vi "main.vi"() -> ()   [LabVIEW 2016]
uses:
  controls/Level2.ctl
panel:
  in  "StringArray":string[](array[string])
  in  "BooleanArray":bool[](array[boolean])
  in  "NumericArray":dbl[](array[numeric])
  in  "BigCluster":T2
  in  "Cluster":T3
  in  "String":string
  in  "Boolean":bool
  in  "Numeric":dbl
  in  "Tab Control":T4(tab)
  in  "BigCluster":T2
  in  "Cluster":T3
  in  "String":string
  in  "Boolean":bool
  in  "Numeric":dbl
  in  "Time lapse(sec)":u32
  in  "Panel Name":string
  in  "Refresh":bool
  in  "Listbox":i32(listbox)
  in  "Panel Name 2":string
  in  "Listbox 2":i32(listbox)
  in  "Run":bool
  in  "DisableListbox":i32(listbox)
  in  "MultiselectListbox":i32[](listbox)
  in  "Single Listbox":i32(listbox)
  out "Listbox Value":i32
  out "Selected Value":i32[](array[numeric])
  in  "Disabled MC Listbox":i32(listbox)
  in  "Multiselect MC Listbox":i32[](listbox)
  in  "MC Listbox":i32(listbox)
  out "MCListbox Value":i32
  out "MCL Selected Value":i32[](array[numeric])
  in  "OK":bool
  in  "Stop":bool
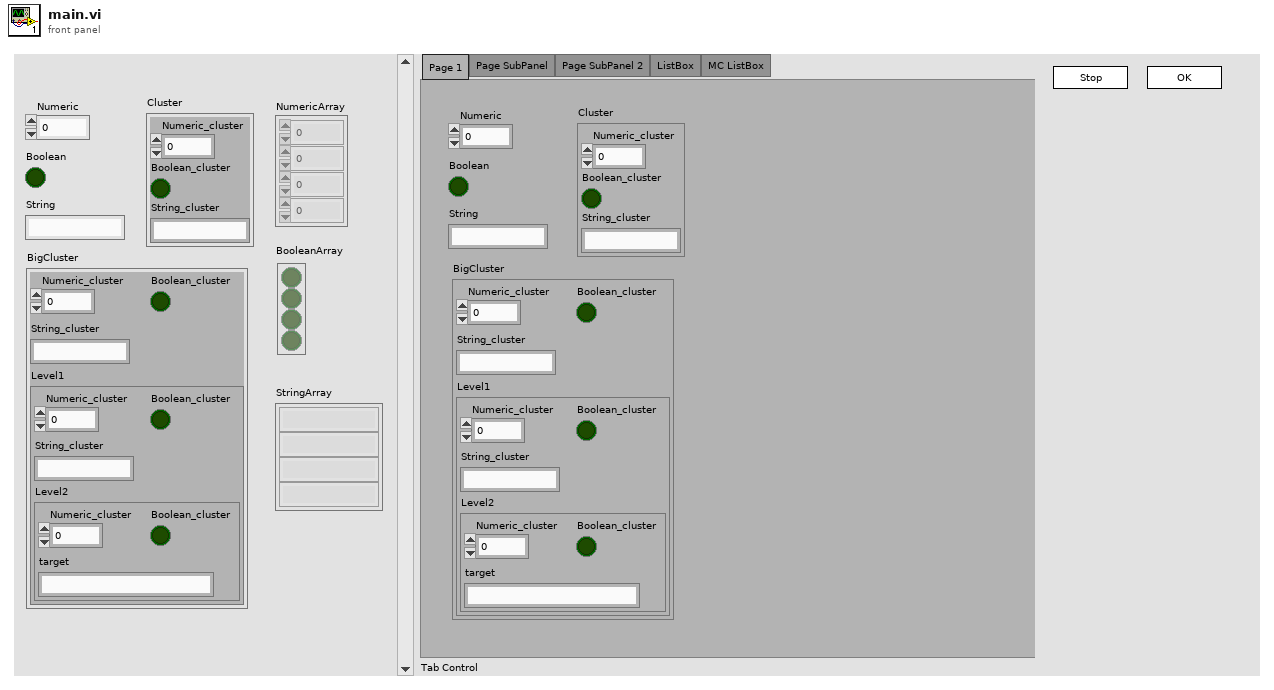
[diagram p1: front panel]
types:
  T1 = typedef "Level2.ctl" = cluster{"Numeric_cluster":dbl, "Boolean_cluster":bool, "target":string}
  T2 = cluster{"Numeric_cluster":dbl, "Boolean_cluster":bool, "String_cluster":string, "Level1":cluster{"Numeric_cluster":dbl, "Boolean_cluster":bool, "String_cluster":string, "Level2":T1}}
  T3 = cluster{"Numeric_cluster":dbl, "Boolean_cluster":bool, "String_cluster":string}
  T4 = enum32{"Page 1", "Page SubPanel", "Page SubPanel 2", "ListBox", "MC ListBox"}
  T5 = enum32{"Invalid", "Standard", "Closed", "Hidden", "Minimized", "Maximized"}
  T6 = enum32{"invalid app kind", "Development System", "Run Time System", "Student Edition", "Embedded LabVIEW", "Evaluation", "Custom"}
  T7 = enum8{"Enabled", "Disabled", "Disabled and Grayed Out"}
  T8 = cluster{"Core":cluster{"Current VI Reference":refnum<vi>, "Close Panel on Exit?":bool}, "VI Name":string, "VI Ref":refnum<vi>, "Panel Folder Path":path, "Time lapse(sec)":u32, "Panel 2 Folder Path":path, "Panel 2 VI ref":refnum<vi>, "VI Running?":bool}
  T9 = cluster{"Current VI Reference":refnum<vi>, "Close Panel on Exit?":bool}
  T10 = enum32{"Bad", "Idle", "Run top level", "Running"}[]
  T11 = enum32{"Bad", "Idle", "Run top level", "Running"}
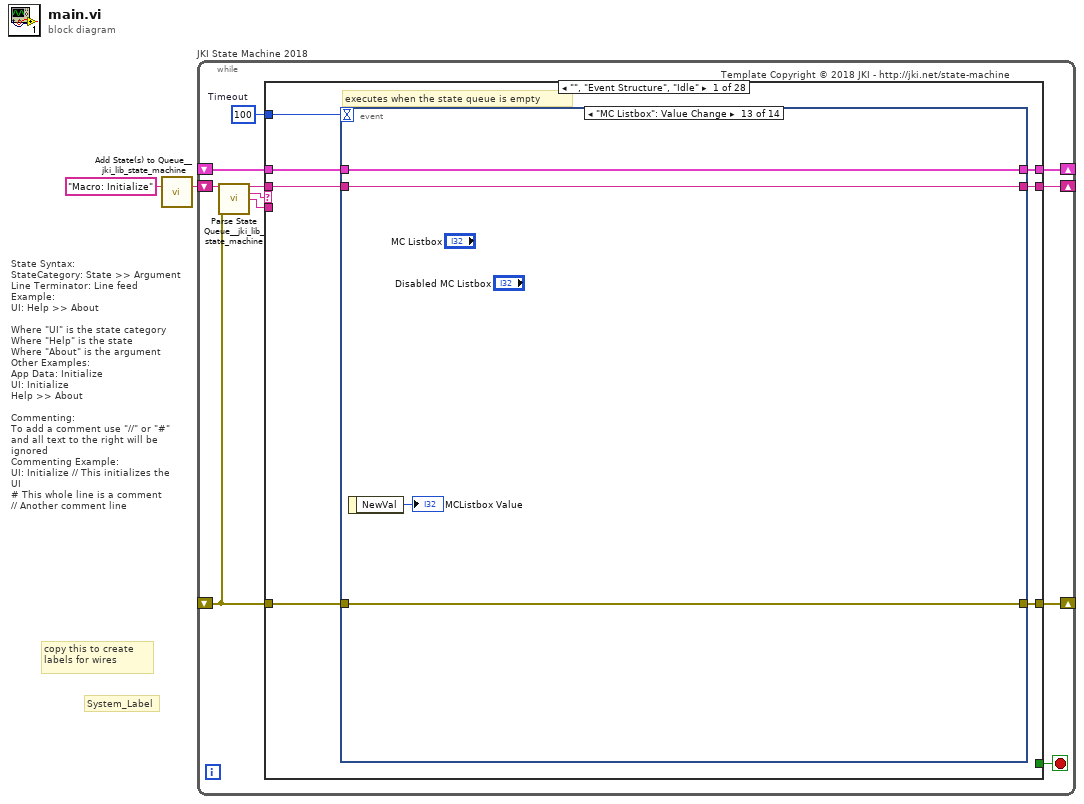
[diagram p0: block diagram]
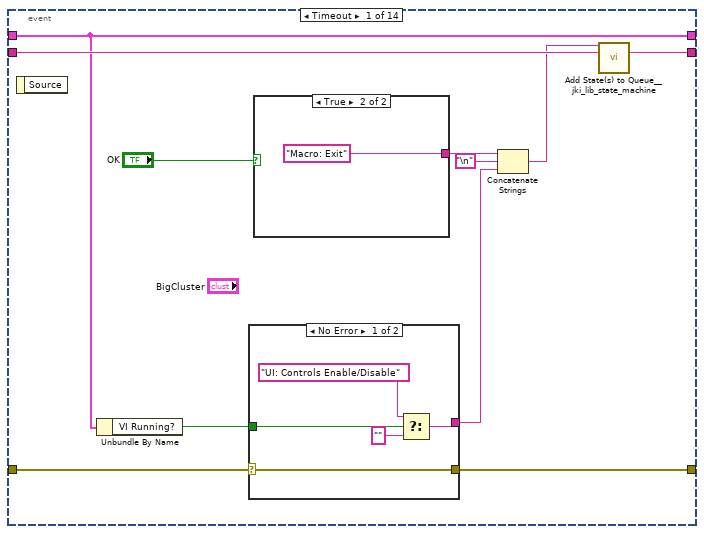
[diagram p2: hidden frame]
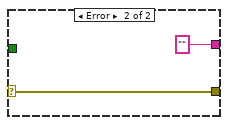
[diagram p3: hidden frame]
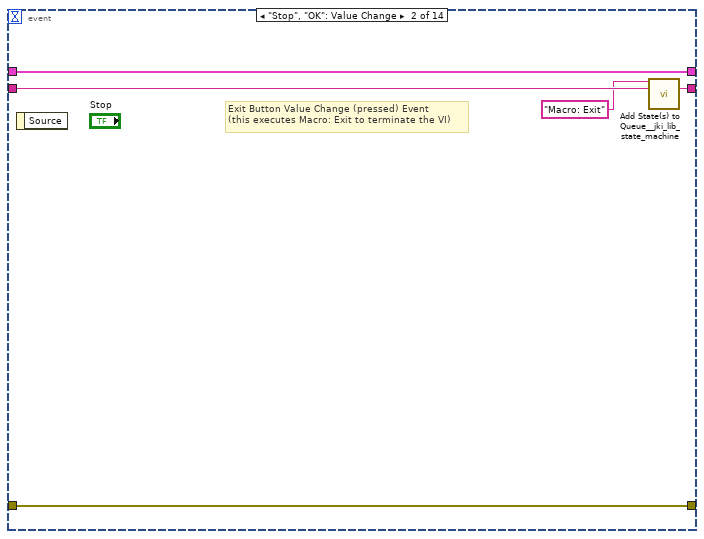
[diagram p5: hidden frame]
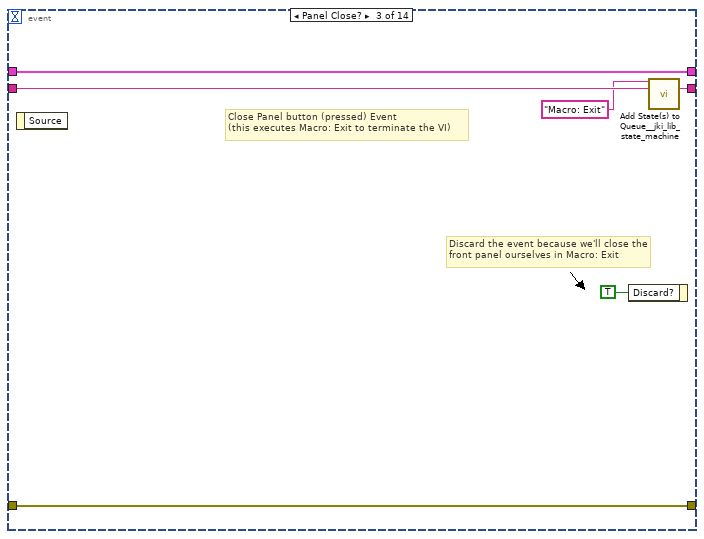
[diagram p6: hidden frame]
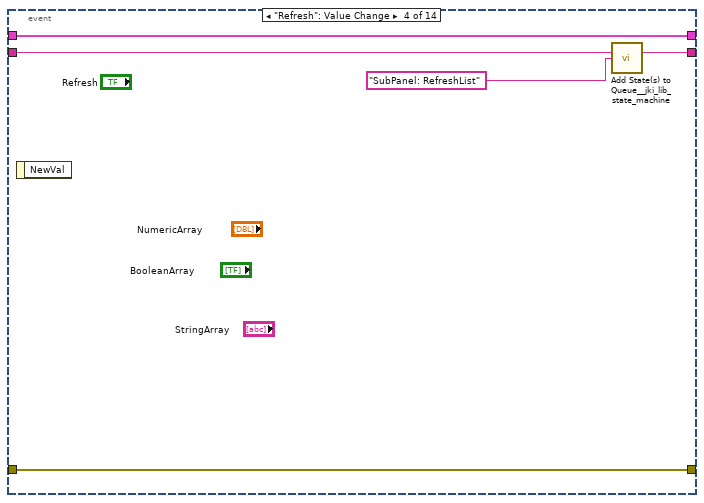
[diagram p7: hidden frame]
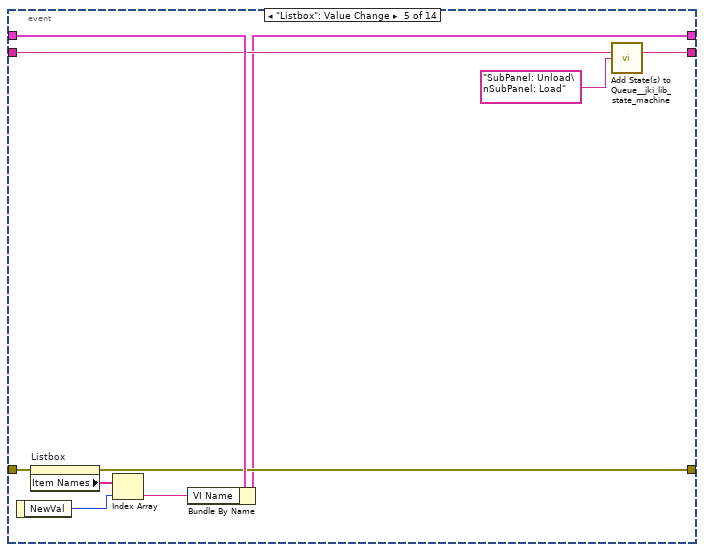
[diagram p8: hidden frame]
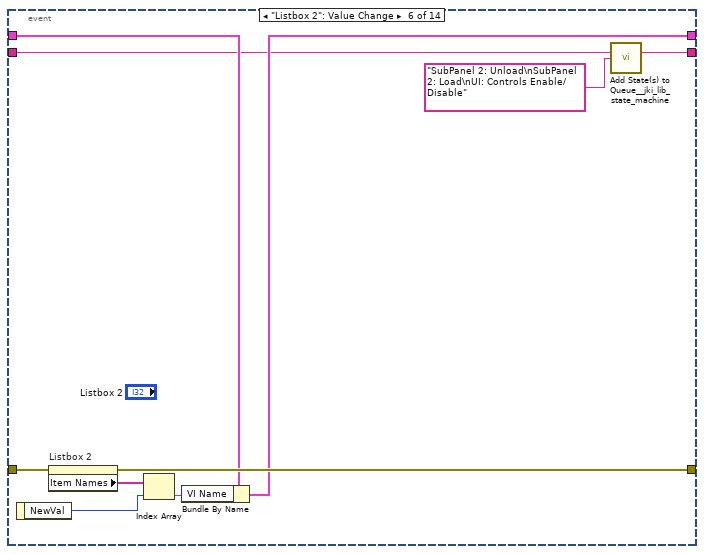
[diagram p9: hidden frame]
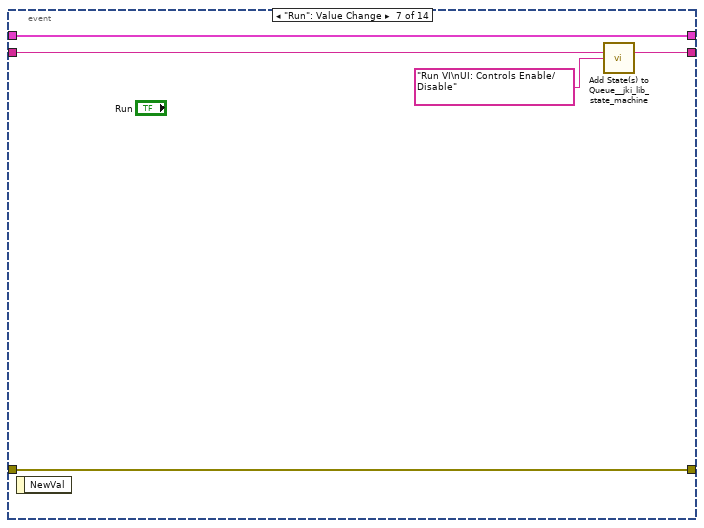
[diagram p10: hidden frame]
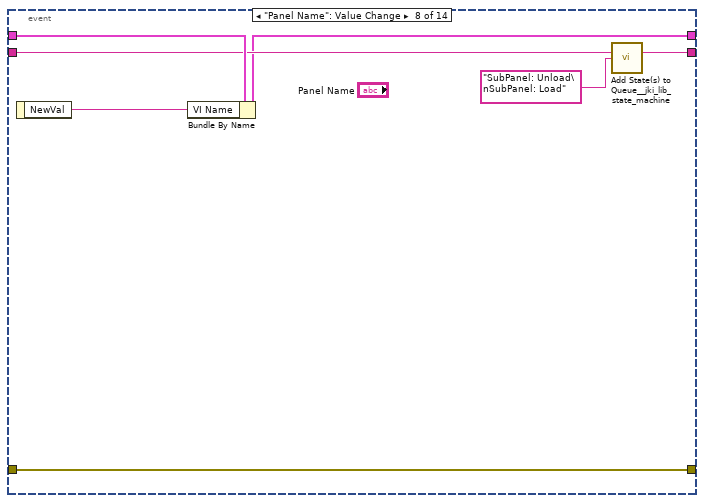
[diagram p11: hidden frame]
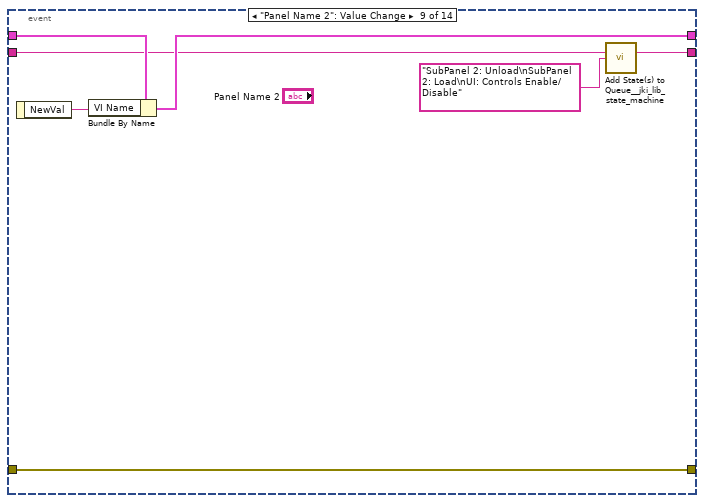
[diagram p12: hidden frame]
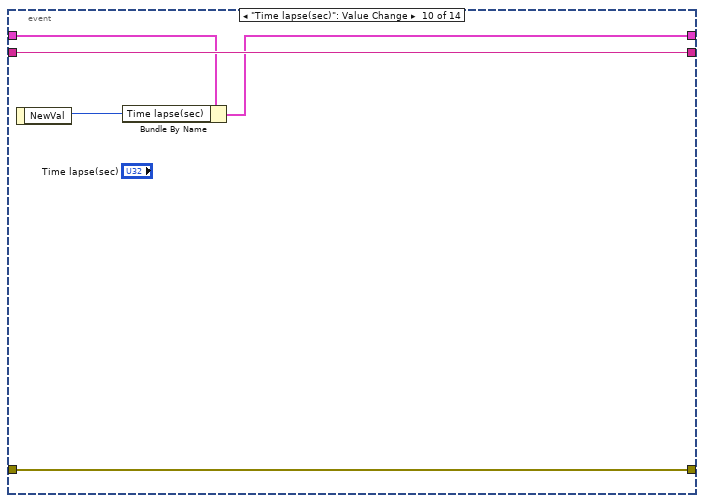
[diagram p13: hidden frame]
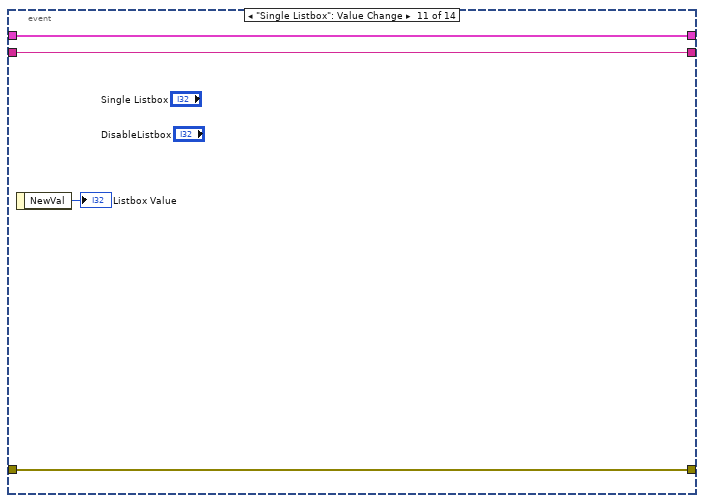
[diagram p14: hidden frame]
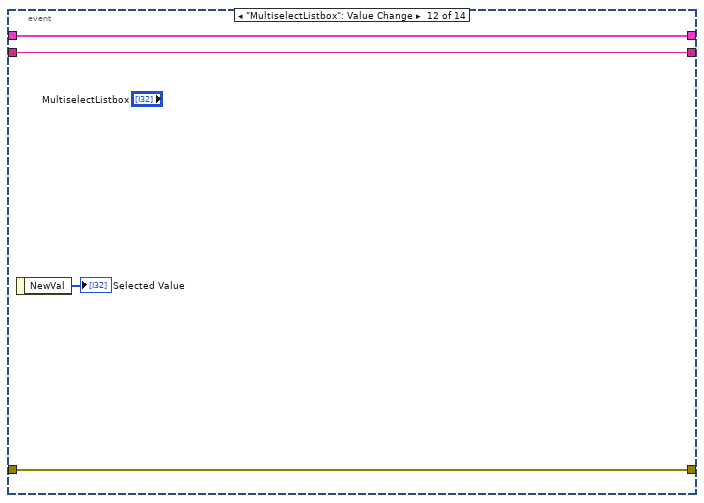
[diagram p15: hidden frame]
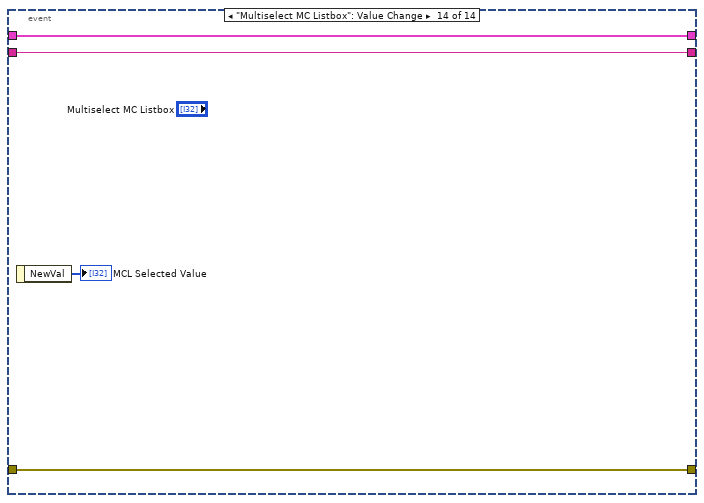
[diagram p16: hidden frame]
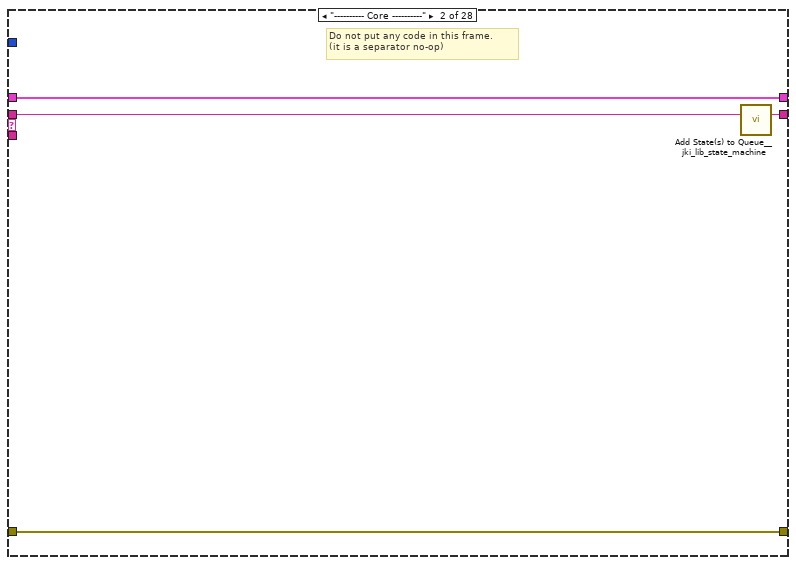
[diagram p17: hidden frame]
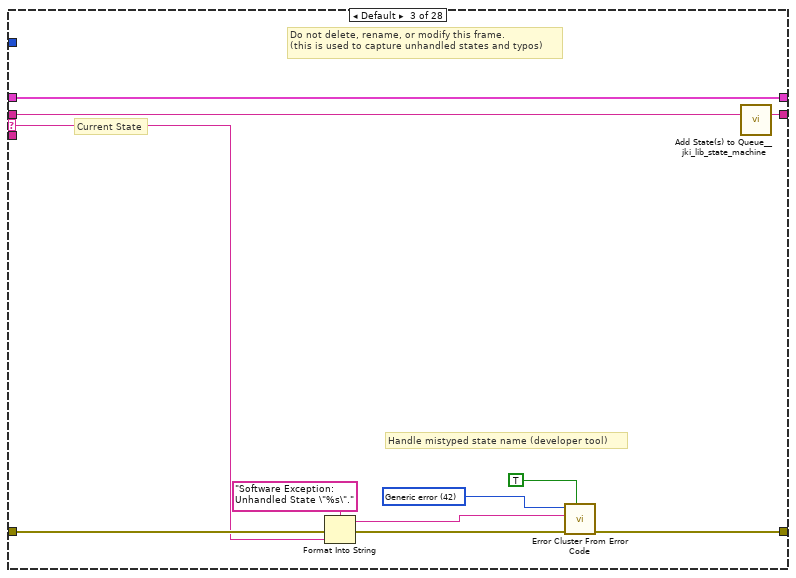
[diagram p18: hidden frame]
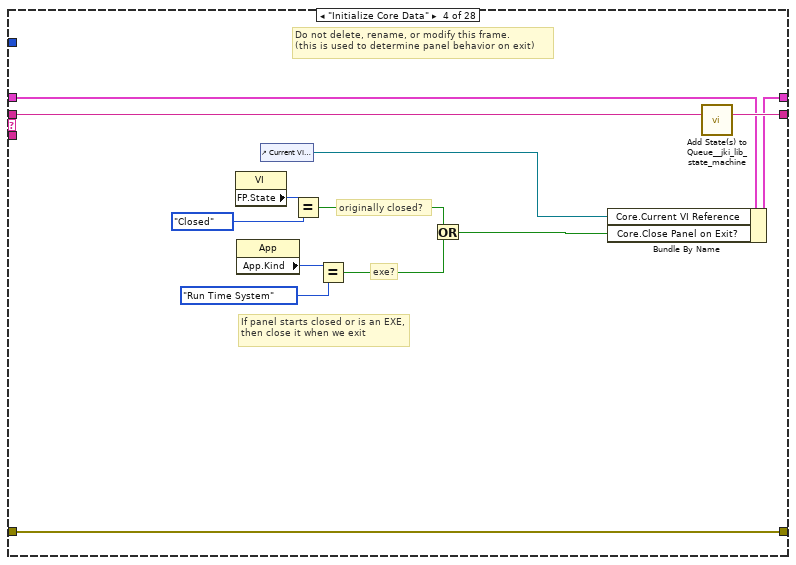
[diagram p19: hidden frame]
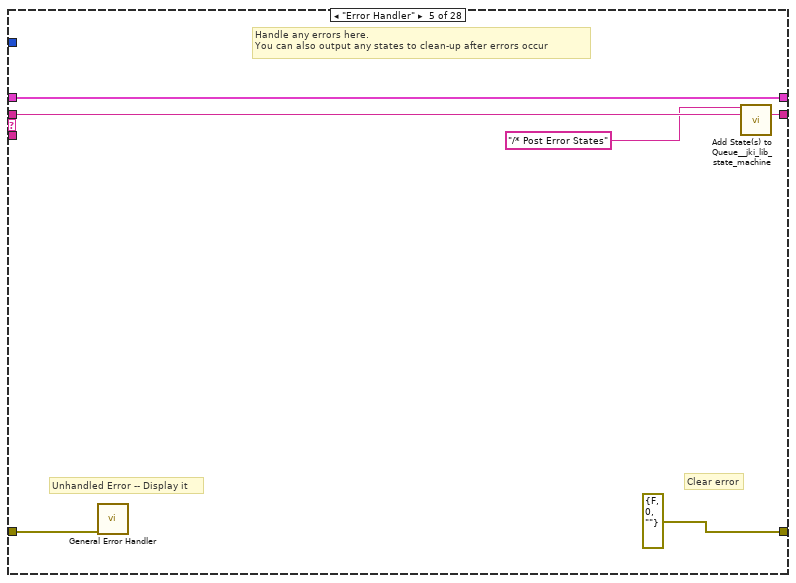
[diagram p20: hidden frame]
diagram:
  # "State Syntax:\nStateCategory: State >> Argument\nLine Terminator: Line feed\nExample:\nUI: Help >> About\n\nWhere \"UI\" is the state category\nWhere \"Help\" is the state\nWhere \"About\" is the argument\nOther Examples:\nApp Data: Initialize\nUI: Initialize\nHelp >> About\n\nCommenting:\nTo add a comment use \"//\" or \"#\" and all text to the right will be ignored\nCommenting Example:\nUI: Initialize // This initializes the UI\n# This whole line is a comment\n// Another comment line"
  # "copy this to create labels for wires"
  # "System_Label"
  n1 = call <vilib>:"Add State(s) to Queue__jki_lib_state_machine.vi"("State(s) in (\"\")"="Macro: Initialize") -> ("States Out"=w2:string)  [unwired: 14 in]
  n2 = while "JKI State Machine 2018" {
    shift-right: [w6] -> _
    shift-left: _ -> [w5]
    shift-right: [w9] -> _
    shift-left: _ -> [w3]
    shift-right: [w8] -> _
    shift-left: w2 -> [w10]
    stop <- w7 stop-if-true
    w4 = 100  # Timeout
    # "Template Copyright © 2018 JKI - http://jki.net/state-machine"
    n3 = call <vilib>:"Parse State Queue__jki_lib_state_machine.vi"("State Queue"=w10, "Error In (no error)"=w3) -> ("Remaining States"=w12:string, "Current State"=w13:string, "Arguments"=w11:string)  [unwired: 11 in]
    n4 = case shown="\"\", \"Event Structure\", \"Idle\"" w13 {
      selector: w13 -> [_ _ w120 _ _ _ _ _ _ _ _ _ _ _ _ _ _ _ _ _ _ _ _ _ _ _ _ _]
      tunnel: w12 -> [w20 w119 w124 w143 w149 w154 w158 w178 w184 w188 w195 w201 w212 w281 w293 w305 w310 w320 w324 w338 w348 w371 w404 w418 w420 w431 w435 w439]
      tunnel: w11 -> [_ _ _ _ _ _ _ _ _ _ _ w196 w206 _ _ _ _ _ _ _ _ _ _ _ _ _ _ _]
      tunnel: w5 -> [w18 w116 w122 w136 w146 w152 w155 _ w179 w185 w193 w199 w208 w279 w283 w302 w307 w317 w321 w333 w345 w366 w402 w410 w419 w424 w432 w436]
      tunnel: [w17 w117 w126 w140 errorcluster {"status"=FALSE, "code"=0, "source"=""} ("error out") w151 w156 w159 w180 w186 w190 w197 w209 w278 w284 w303 w308 w318 w322 w326 w339 w369 w400 w412 w421 w426 w433 w437] -> w9
      tunnel: w3 -> [w16 w117 w125 w140 w145 w151 w156 w160 w181 w186 w192 w198 w210 w278 w285 w303 w308 w318 w322 w336 w341 w363 w403 w413 w421 w429 w433 w437]
      tunnel: [w19 w118 w123 w142 w148 w153 w157 w177 w183 w187 w194 w200 w211 w280 w293 w304 w309 w319 w323 w337 w347 w370 w404 w418 w420 w431 w434 w438] -> w8
      tunnel: [_ _ _ _ _ TRUE _ _ _ _ _ _ _ _ _ _ _ _ _ _ _ _ _ _ _ _ _ _] -> w7
      tunnel: [w15 w116 w122 w141 w146 w152 w155 w172 w179 w185 w193 w199 w208 w279 w283 w302 w307 w317 w321 w333 w345 w365 w402 w409 w419 w423 w432 w436] -> w6
      tunnel: w4 -> [w14 _ _ _ _ _ _ _ _ _ _ _ _ _ _ _ _ _ _ _ _ _ _ _ _ _ _ _]
      frame "", "Event Structure", "Idle" {
        # "executes when the state queue is empty"
        n5 = event shown="[12] \"MC Listbox\": Value Change" {
          selector: _ -> [_ _ _ _ _ _ _ _ _ _ _ _ _ _]
          dyn-events: _ -> [_ _ _ _ _ _ _ _ _ _ _ _ _ _]
          timeout: w14 -> [_ _ _ _ _ _ _ _ _ _ _ _ _ _]
          tunnel: w20 -> [w31 w44 w50 w53 w64 w67 w78 w86 w89 w99 w103 w107 w111 w115]
          tunnel: [w30 w43 w49 w52 w63 w66 w77 w85 w88 w99 w103 w107 w111 w115] -> w19
          tunnel: w18 -> [w28 w41 w47 w54 w65 w70 w79 w87 w92 w96 w101 w105 w109 w113]
          tunnel: [w21 w42 w48 w55 w60 w73 w80 w83 w94 w98 w102 w106 w110 w114] -> w17
          tunnel: w16 -> [w22 w42 w48 w55 w61 w74 w80 w83 w94 w98 w102 w106 w110 w114]
          tunnel: [w28 w41 w47 w54 w57 w69 w79 w81 w91 w95 w101 w105 w109 w113] -> w15
          event Timeout {
            n6 = event-data() -> ()  [unwired: 1 in, 1 out]
            n7 = Unbundle By Name(w28) -> ("VI Running?"=w27:bool)
            n8 = case shown="No Error" w22 {
              selector: w22 -> [w32 w37]
              tunnel: [w33 ""] -> w26
              tunnel: w27 -> [w36 _]
              tunnel: [w32 w37] -> w21
              frame No Error {
                n9 = Select(t="UI: Controls Enable/Disable", s=w36, f="") -> (s? t:f=w33:string)
              }
              frame Error {
              }
            }
            n10 = case shown="True" "OK" {
              tunnel: [_ "Macro: Exit"] -> w25
              frame False {
              }
              frame True {
              }
            }
            n11 = Concatenate Strings(w25, "\n", w26) -> (w23:string)
            n12 = call <vilib>:"Add State(s) to Queue__jki_lib_state_machine.vi"("State(s) in Front (\"\")"=w23, "State(s) in (\"\")"=w31) -> ("States Out"=w30:string)  [unwired: 13 in]
          }
          event "Stop", "OK": Value Change {
            # "Exit Button Value Change (pressed) Event\n(this executes Macro: Exit to terminate the VI)"
            n13 = event-data() -> ()  [unwired: 1 in, 1 out]
            n14 = call <vilib>:"Add State(s) to Queue__jki_lib_state_machine.vi"("State(s) in Front (\"\")"="Macro: Exit", "State(s) in (\"\")"=w44) -> ("States Out"=w43:string)  [unwired: 13 in]
          }
          event Panel Close? {
            # "Discard the event because we'll close the front panel ourselves in Macro: Exit"
            # "Close Panel button (pressed) Event\n(this executes Macro: Exit to terminate the VI)"
            n15 = event-data() -> ()  [unwired: 1 in, 1 out]
            n16 = event-data("Discard?"=TRUE) -> ()  [unwired: 1 in, 1 out]
            n17 = call <vilib>:"Add State(s) to Queue__jki_lib_state_machine.vi"("State(s) in Front (\"\")"="Macro: Exit", "State(s) in (\"\")"=w50) -> ("States Out"=w49:string)  [unwired: 13 in]
          }
          event "Refresh": Value Change {
            n18 = event-data() -> ()  [unwired: 1 in, 1 out]
            n19 = call <vilib>:"Add State(s) to Queue__jki_lib_state_machine.vi"("State(s) in (\"\")"=w53, "State(s) at Back (\"\")"="SubPanel: RefreshList") -> ("States Out"=w52:string)  [unwired: 13 in]
          }
          event "Listbox": Value Change {
            n20 = event-data() -> ("NewVal"=w58:i32)  [unwired: 1 in]
            n21 = property on="Listbox" class="LstBox (strict)"(error in=w61) -> (error out=w60:errorcluster, "Item Names"=w59:string[])  [unwired: 1 in, 1 out]
            n22 = Index Array(array=w59, index=w58) -> (element=w56:string)
            n23 = Bundle By Name(cluster=w65, "VI Name"=w56) -> (w57:T8)
            n24 = call <vilib>:"Add State(s) to Queue__jki_lib_state_machine.vi"("State(s) in (\"\")"=w64, "State(s) at Back (\"\")"="SubPanel: Unload\nSubPanel: Load") -> ("States Out"=w63:string)  [unwired: 13 in]
          }
          event "Listbox 2": Value Change {
            n25 = event-data() -> ("NewVal"=w72:i32)  [unwired: 1 in]
            n26 = property on="Listbox 2" class="LstBox (strict)"(error in=w74) -> (error out=w73:errorcluster, "Item Names"=w75:string[])  [unwired: 1 in, 1 out]
            n27 = Index Array(array=w75, index=w72) -> (element=w71:string)
            n28 = Bundle By Name(cluster=w70, "VI Name"=w71) -> (w69:T8)
            n29 = call <vilib>:"Add State(s) to Queue__jki_lib_state_machine.vi"("State(s) in (\"\")"=w67, "State(s) at Back (\"\")"="SubPanel 2: Unload\nSubPanel 2: Load\nUI: Controls Enable/Disable") -> ("States Out"=w66:string)  [unwired: 13 in]
          }
          event "Run": Value Change {
            n30 = event-data() -> ()  [unwired: 1 in, 1 out]
            n31 = call <vilib>:"Add State(s) to Queue__jki_lib_state_machine.vi"("State(s) in (\"\")"=w78, "State(s) at Back (\"\")"="Run VI\nUI: Controls Enable/Disable" ("State(s) at Back (\"\")")) -> ("States Out"=w77:string)  [unwired: 13 in]
          }
          event "Panel Name": Value Change {
            n32 = event-data() -> ("NewVal"=w82:string)  [unwired: 1 in]
            n33 = Bundle By Name(cluster=w87, "VI Name"=w82) -> (w81:T8)
            n34 = call <vilib>:"Add State(s) to Queue__jki_lib_state_machine.vi"("State(s) in (\"\")"=w86, "State(s) at Back (\"\")"="SubPanel: Unload\nSubPanel: Load") -> ("States Out"=w85:string)  [unwired: 13 in]
          }
          event "Panel Name 2": Value Change {
            n35 = event-data() -> ("NewVal"=w93:string)  [unwired: 1 in]
            n36 = Bundle By Name(cluster=w92, "VI Name"=w93) -> (w91:T8)
            n37 = call <vilib>:"Add State(s) to Queue__jki_lib_state_machine.vi"("State(s) in (\"\")"=w89, "State(s) at Back (\"\")"="SubPanel 2: Unload\nSubPanel 2: Load\nUI: Controls Enable/Disable") -> ("States Out"=w88:string)  [unwired: 13 in]
          }
          event "Time lapse(sec)": Value Change {
            n38 = event-data() -> ("NewVal"=w97:u32)  [unwired: 1 in]
            n39 = Bundle By Name(cluster=w96, "Time lapse(sec)"=w97) -> (w95:T8)
          }
          event "Single Listbox": Value Change {
            n40 = event-data() -> ("NewVal"=→"Listbox Value":i32)  [unwired: 1 in]
          }
          event "MultiselectListbox": Value Change {
            n41 = event-data() -> ("NewVal"=→"Selected Value":i32[])  [unwired: 1 in]
          }
          event "MC Listbox": Value Change {
            n42 = event-data() -> ("NewVal"=→"MCListbox Value":i32)  [unwired: 1 in]
          }
          event "Multiselect MC Listbox": Value Change {
            n43 = event-data() -> ("NewVal"=→"MCL Selected Value":i32[])  [unwired: 1 in]
          }
        }
      }
      frame "---------- Core ----------" {
        # "Do not put any code in this frame.\n(it is a separator no-op)"
        n44 = call <vilib>:"Add State(s) to Queue__jki_lib_state_machine.vi"("State(s) in (\"\")"=w119) -> ("States Out"=w118:string)  [unwired: 14 in]
      }
      frame Default {
        w129 = 42 items=["No error", "Argument error", "Memory is full", "Out of zone", "End of file", "File already open", "Generic file I/O error", "File not found", "File permission error", "Disk is full", "Duplicate path", "Too many files open", "System feature not enabled", "Resource file not found", "Cannot add resource", "Resource not found", "Image not found", "Image memory error", "Pen does not exist", "Config type invalid", "Config token not found", "Config parse error", "Config memory error", "Bad external code format", "Bad external code offset", "External code not present", "Null window", "Destroy window error", "Null menu", "Print aborted", "Bad print record", "Print driver error", "Windows error during printing", "Memory error during printing", "Print dialog error", "Generic print error", "Invalid device refnum", "Device not found", "Device parameter error", "Device unit error", "Cannot open device", "Device call aborted", "Generic error", "Cancelled by user", "Object ID too low", "Object ID too high", "Object not in heap", "Unknown heap", "Unknown object (invalid DefProc)", "Unknown object (DefProc not in table)", "Message out of range", "Invalid (null) method", "Unknown message", "Manager call not supported", "Bad address", "Network operation in progress", "Network operation timed out", "Connection is busy", "Network attribute not supported", "Network error", "Address in use", "System out of memory", "Connection aborted", "Connection refused", "Not connected", "Already connected", "Connection closed", "Initialization error (interapplication manager)", "Bad occurrence", "Wait on unbound occurrence handler", "Occurrence queue overflow", "Datalog type conflict", "Unused", "Unrecognized type (interapplication manager)", "Memory corrupt", "Failed to make temporary DLL", "Old CIN version", "Drag socket not found", "Failed to load drop-object", "Failed to register OLE object", "Failed to release OLE object", "Format specifier type mismatch", "Unknown format specifier", "Too few format specifiers", "Too many format specifiers", "Scan failed", "Newer CIN version", "Error converting to variant", "Runtime menu error", "Password tampered", "Variant attribute not found", "Incompatible variant data type", "Event data is not available", "Event Store is not present", "Occurrence is not found", "Event Queue is not created", "Event info is not available", "Refnum passed is NULL", "Error retrieving Class GUID", "Error retrieving CoClass GUID", "Error retrieving TypeLib GUID.", "Bad built application magic bytes.", "Specific driver is different from the specific driver associated with the Logical Name.", "There is no session opened to the class driver.", "Max Error", "MAX - Error with config objects", "MAX - Error loading configuration", "MAX - Group not supported"]
        # "Current State"
        # "Do not delete, rename, or modify this frame.\n(this is used to capture unhandled states and typos)"
        # "Handle mistyped state name (developer tool)"
        n45 = Format Into String(format string="Software Exception: Unhandled State \"%s\"." ("message"), error in=w125, w120) -> (resulting string=w128:string, error out=w127:errorcluster)  [unwired: 1 in]
        n46 = call <vilib>:"Error Cluster From Error Code.vi"("show call chain? (False)"=TRUE, "error in (no error)"=w127, "error message (\"\")"=w128, "error code (0)"=w129) -> ("error out"=w126:errorcluster)  [unwired: 5 in]
        n47 = call <vilib>:"Add State(s) to Queue__jki_lib_state_machine.vi"("State(s) in (\"\")"=w124) -> ("States Out"=w123:string)  [unwired: 14 in]
      }
      frame "Initialize Core Data" {
        # "Do not delete, rename, or modify this frame.\n(this is used to determine panel behavior on exit)"
        # "originally closed?"
        # "exe?"
        # "If panel starts closed or is an EXE, then close it when we exit"
        n48 = property class="VI"() -> ("FP.State"=w133:T5)  [unwired: 2 in, 2 out]
        n49 = property class="App"() -> ("App.Kind"=w139:T6)  [unwired: 2 in, 2 out]
        n50 = control-ref of="Current VI Reference"() -> (w134:refnum<vi>)
        n51 = Equal?(x=w133, y=T5."Closed" ("Front Panel Window:State")) -> (x = y?=w131:bool)
        n52 = Equal?(x=w139, y=T6."Run Time System" ("Application:Kind")) -> (x = y?=w137:bool)
        n53 = Or(x=w131, y=w137) -> (x .or. y?=w135:bool)
        n54 = Bundle By Name(cluster=w136, "Core.Current VI Reference"=w134, "Core.Close Panel on Exit?"=w135) -> (w141:T8)
        n55 = call <vilib>:"Add State(s) to Queue__jki_lib_state_machine.vi"("State(s) in (\"\")"=w143) -> ("States Out"=w142:string)  [unwired: 14 in]
      }
      frame "Error Handler" {
        # "Unhandled Error -- Display it"
        # "Handle any errors here.\nYou can also output any states to clean-up after errors occur"
        # "Clear error"
        n56 = call <vilib>:"General Error Handler.vi"("error in (no error)"=w145) -> ()  [unwired: 10 in, 5 out]
        n57 = call <vilib>:"Add State(s) to Queue__jki_lib_state_machine.vi"("State(s) in Front (\"\")"="/* Post Error States", "State(s) in (\"\")"=w149) -> ("States Out"=w148:string)  [unwired: 13 in]
      }
      frame "Exit" {
        # "Do not put any code in this frame.\n(No errors that occur here will be handled.)"
        n58 = call <vilib>:"Add State(s) to Queue__jki_lib_state_machine.vi"("State(s) in (\"\")"=w154) -> ("States Out"=w153:string)  [unwired: 14 in]
      }
      frame "---------- Data ----------" {
        # "Do not put any code in this frame.\n(It is a separator no-op. You can make a copy of this frame to create a new Data frame)"
        n59 = call <vilib>:"Add State(s) to Queue__jki_lib_state_machine.vi"("State(s) in (\"\")"=w158) -> ("States Out"=w157:string)  [unwired: 14 in]
      }
      frame "Data: Initialize" {
        w166 = FALSE  # VI Running?
        w167 = refnum<vi> refnum  # Panel 2 VI ref
        w169 = path ""  # Panel 2 Folder Path
        w170 = u32 0  # Time lapse(sec)
        w171 = refnum<vi> refnum  # VI Ref
        w173 = path ""  # Panel Folder Path
        w174 = T9 {"Current VI Reference"=refnum, "Close Panel on Exit?"=FALSE}  # Core
        w175 = ""  # VI Name
        # "Initialize the shift-register data, here.\n(data names are defined by what you wire into the bundle function)"
        n60 = vi-ref "_Template.vi"() -> (w163:refnum<vi>)
        n61 = property class="VI"(reference=w163, error in=w160) -> (error out=w159:errorcluster, "Path"=w162:path)  [unwired: 1 out]
        n62 = Strip Path(path=w162) -> (stripped path=w161:path)  [unwired: 1 out]
        n63 = Bundle("Core"=w174, "VI Name"=w175, "VI Ref"=w171, "Panel Folder Path"=w173, "Time lapse(sec)"=w170, "Panel 2 Folder Path"=w169, "Panel 2 VI ref"=w167, "VI Running?"=w166) -> (w176:T8)  [unwired: 1 in]
        n64 = Strip Path(path=w161) -> (stripped path=w165:path)  [unwired: 1 out]
        n65 = Build Path(base path=w165, name or relative path="ExecPanels") -> (appended path=w168:path)
        n66 = Bundle By Name(cluster=w176, "Panel Folder Path"=w161, "Panel 2 Folder Path"=w168) -> (w172:T8)
        n67 = call <vilib>:"Add State(s) to Queue__jki_lib_state_machine.vi"("State(s) in (\"\")"=w178) -> ("States Out"=w177:string)  [unwired: 14 in]
      }
      frame "Data: Cleanup" {
        # "Cleanup any data and references, here.\n(this is called automatically, by the Macro: Exit)"
        n68 = Unbundle By Name(w179) -> ("Core.Current VI Reference"=w182:refnum<vi>)
        n69 = Close Reference(reference=w182, error in (no error)=w181) -> (error out=w180:errorcluster)
        n70 = call <vilib>:"Add State(s) to Queue__jki_lib_state_machine.vi"("State(s) in (\"\")"=w184) -> ("States Out"=w183:string)  [unwired: 14 in]
      }
      frame "---------- UI ----------" {
        # "Do not put any code in this frame.\n(It is a separator no-op. You can make a copy of this frame to create a new UI frame)"
        n71 = call <vilib>:"Add State(s) to Queue__jki_lib_state_machine.vi"("State(s) in (\"\")"=w188) -> ("States Out"=w187:string)  [unwired: 14 in]
      }
      frame "UI: Initialize" {
        # "Initialize the User Interface, here.\n(this is called automatically, by the Macro: Init)"
        n72 = invoke class="VI" method="Default Vals.Reinit All"(error in=w192) -> (error out=w191:errorcluster)  [unwired: 2 in, 2 out]
        n73 = property on="Run" class="Bool"(error in=w191, "DisabledEnum"=T7."Disabled and Grayed Out" ("Disabled")) -> (error out=w190:errorcluster)  [unwired: 1 in, 1 out]
        n74 = call <vilib>:"Add State(s) to Queue__jki_lib_state_machine.vi"("State(s) in (\"\")"=w195) -> ("States Out"=w194:string)  [unwired: 14 in]
      }
      frame "UI: Cursor Set" {
        # "Argument"
        # "Set and Unset Cursor Busy.\n(Usage: \"UI: Cursor Set >> Busy|Idle\")"
        n75 = case shown="\"Idle\", Default" w196 {
          tunnel: w198 -> [w203 w205]
          tunnel: [w202 w204] -> w197
          frame "Idle", Default {
            n76 = call <vilib>:"Unset Busy.vi"("error in (no error)"=w203) -> ("error out"=w202:errorcluster)  [unwired: 10 in]
          }
          frame "Busy" {
            n77 = call <vilib>:"Set Busy.vi"("error in (no error)"=w205) -> ("error out"=w204:errorcluster)  [unwired: 9 in, 1 out]
          }
        }
        n78 = call <vilib>:"Add State(s) to Queue__jki_lib_state_machine.vi"("State(s) in (\"\")"=w201) -> ("States Out"=w200:string)  [unwired: 14 in]
      }
      frame "UI: Front Panel State" {
        # "Argument"
        # "Set Front Panel Open or Closed\n(Usage: \"UI: Front Panel State >> Open|Close\")"
        n79 = Unbundle By Name(w208) -> ("Core.Current VI Reference"=w207:refnum<vi>)
        n80 = case shown="\"Close\", \"Closed\"" w206 {
          tunnel: w210 -> [w218 w233 w244 w257 w270]
          tunnel: [w220 w234 w246 w259 w272] -> w209
          tunnel: w207 -> [w219 w231 w245 w258 w271]
          frame "Open", "Standard", Default {
            w213 = T5."Standard" ("State")
            n81 = property class="VI"(reference=w219, error in=w218) -> (reference out=w216:refnum<vi>, error out=w217:errorcluster, "FP.State"=w215:T5)
            n82 = Not Equal?(x=w215, y=w213) -> (x != y?=w214:bool)
            n83 = case shown="True" w214 {
              tunnel: [w224 w226] -> w220
              tunnel: w217 -> [w223 w226]
              tunnel: w216 -> [w222 _]
              tunnel: w213 -> [w221 _]
              frame True {
                n84 = invoke class="VI" method="FP.Open"(reference=w222, error in=w223, "Activate"=TRUE, "State"=w221) -> (error out=w224:errorcluster)  [unwired: 1 in, 4 out]
              }
              frame False {
              }
            }
          }
          frame "Close", "Closed" {
            n85 = property class="VI"(reference=w231, error in=w233) -> (reference out=w230:refnum<vi>, error out=w232:errorcluster, "FP.State"=w228:T5)
            n86 = Not Equal?(x=w228, y=T5."Closed" ("Front Panel Window:State")) -> (x != y?=w227:bool)
            n87 = case shown="True" w227 {
              tunnel: [w235 w238] -> w234
              tunnel: w232 -> [w235 w237]
              tunnel: w230 -> [_ w236]
              frame False {
              }
              frame True {
                n88 = invoke class="VI" method="FP.Close"(reference=w236, error in=w237) -> (error out=w238:errorcluster)  [unwired: 1 in, 2 out]
              }
            }
          }
          frame "Hidden", "Hide" {
            w239 = T5."Hidden" ("State")
            n89 = property class="VI"(reference=w245, error in=w244) -> (reference out=w242:refnum<vi>, error out=w243:errorcluster, "FP.State"=w241:T5)
            n90 = Not Equal?(x=w241, y=w239) -> (x != y?=w240:bool)
            n91 = case shown="True" w240 {
              tunnel: [w250 w251] -> w246
              tunnel: w243 -> [w249 w251]
              tunnel: w242 -> [w248 _]
              tunnel: w239 -> [w247 _]
              frame True {
                n92 = invoke class="VI" method="FP.Open"(reference=w248, error in=w249, "State"=w247) -> (error out=w250:errorcluster)  [unwired: 2 in, 4 out]
              }
              frame False {
              }
            }
          }
          frame "Minimize", "Minimized" {
            w252 = T5."Minimized" ("State")
            n93 = property class="VI"(reference=w258, error in=w257) -> (reference out=w255:refnum<vi>, error out=w256:errorcluster, "FP.State"=w254:T5)
            n94 = Not Equal?(x=w254, y=w252) -> (x != y?=w253:bool)
            n95 = case shown="True" w253 {
              tunnel: [w263 w264] -> w259
              tunnel: w256 -> [w262 w264]
              tunnel: w255 -> [w261 _]
              tunnel: w252 -> [w260 _]
              frame True {
                n96 = invoke class="VI" method="FP.Open"(reference=w261, error in=w262, "State"=w260) -> (error out=w263:errorcluster)  [unwired: 2 in, 4 out]
              }
              frame False {
              }
            }
          }
          frame "Maximize", "Maximized" {
            w265 = T5."Maximized" ("State")
            n97 = property class="VI"(reference=w271, error in=w270) -> (reference out=w268:refnum<vi>, error out=w269:errorcluster, "FP.State"=w267:T5)
            n98 = Not Equal?(x=w267, y=w265) -> (x != y?=w266:bool)
            n99 = case shown="True" w266 {
              tunnel: [w276 w277] -> w272
              tunnel: w269 -> [w275 w277]
              tunnel: w268 -> [w274 _]
              tunnel: w265 -> [w273 _]
              frame True {
                n100 = invoke class="VI" method="FP.Open"(reference=w274, error in=w275, "State"=w273) -> (error out=w276:errorcluster)  [unwired: 2 in, 4 out]
              }
              frame False {
              }
            }
          }
        }
        n101 = call <vilib>:"Add State(s) to Queue__jki_lib_state_machine.vi"("State(s) in (\"\")"=w212) -> ("States Out"=w211:string)  [unwired: 14 in]
      }
      frame "UI: Update" {
        n102 = call <vilib>:"Add State(s) to Queue__jki_lib_state_machine.vi"("State(s) in (\"\")"=w281) -> ("States Out"=w280:string)  [unwired: 14 in]
      }
      frame "UI: Controls Enable/Disable" {
        w289 = T10 [enum."Running", enum."Bad", enum."Run top level"] items=["Bad", "Idle", "Run top level", "Running"] ("y")
        n103 = property on="Sub Panel 2" class="SubPnl"(error in=w285) -> (error out=w291:errorcluster, "InsertedVI"=w292:refnum<vi>)  [unwired: 1 in, 1 out]
        n104 = property class="VI"(reference=w292, error in=w291) -> (error out=w286:errorcluster, "Exec.State"=w290:T11)  [unwired: 1 out]
        n105 = Equal?(x=w290, y=w289) -> (x = y?=w288:bool[])
        n106 = Or Array Elements(Boolean array=w288) -> (logical OR=w287:bool)
        n107 = case shown="False" w287 {
          selector: w287 -> [w294 w298]
          tunnel: w286 -> [w296 w301]
          tunnel: [w295 w299] -> w284
          tunnel: [w294 w298] -> w282
          frame False {
            n108 = property on="Run" class="Bool"(error in=w296, "DisabledEnum"=T7."Enabled" ("Disabled")) -> (error out=w295:errorcluster)  [unwired: 1 in, 1 out]
          }
          frame True {
            n109 = property on="Run" class="Bool"(error in=w301, "DisabledEnum"=T7."Disabled and Grayed Out" ("Disabled")) -> (error out=w299:errorcluster)  [unwired: 1 in, 1 out]
          }
        }
        n110 = Bundle By Name(cluster=w283, "VI Running?"=w282) -> ()  [unwired: 1 out]
      }
      frame "---------- Macro ----------" {
        # "Do not put any code in this frame.\n(It is a separator no-op. You can make a copy of this frame to create a new Macro frame)"
        n111 = call <vilib>:"Add State(s) to Queue__jki_lib_state_machine.vi"("State(s) in (\"\")"=w305) -> ("States Out"=w304:string)  [unwired: 14 in]
      }
      frame "Macro: Initialize" {
        w306 = "Data: Initialize\nInitialize Core Data\nUI: Initialize\nUI: Front Panel State >> Open\n# Custom States\nSubPanel: RefreshList"  # Data: Initialize Initialize Core Data UI: Initialize UI: Front Panel State >> Open # Custom States SubPanel: RefreshList
        # "Initialization Macro\n(This is called once, when the VI starts)"
        n112 = call <vilib>:"Add State(s) to Queue__jki_lib_state_machine.vi"("State(s) in Front (\"\")"=w306, "State(s) in (\"\")"=w310) -> ("States Out"=w309:string)  [unwired: 13 in]
      }
      frame "Macro: Exit" {
        # "Exit Macro\n(This is called once, when the VI exits)"
        n113 = Unbundle By Name(w317) -> ("Core.Close Panel on Exit?"=w316:bool)
        n114 = Select(t="UI: Front Panel State >> Close", s=w316, f="") -> (s? t:f=w313:string)
        n115 = call <vilib>:"Add State(s) to Queue__jki_lib_state_machine.vi"("State(s) in (\"\")"=w313, "State(s) at Back (\"\")"="SubPanel: Unload\nSubPanel 2: Unload\nData: Cleanup\nExit") -> ("States Out"=w311:string)  [unwired: 13 in]
        n116 = call <vilib>:"Add State(s) to Queue__jki_lib_state_machine.vi"("State(s) in Front (\"\")"=w311, "State(s) in (\"\")"=w320) -> ("States Out"=w319:string)  [unwired: 13 in]
      }
      frame "---------- SubPanel ----------" {
        # "Template Separator\n(You can make a copy of, or modify, this frame)"
        n117 = call <vilib>:"Add State(s) to Queue__jki_lib_state_machine.vi"("State(s) in (\"\")"=w324) -> ("States Out"=w323:string)  [unwired: 14 in]
      }
      frame "SubPanel: RefreshList" {
        w325 = -1 ("Listbox")
        n118 = Unbundle By Name(w333) -> ("Panel 2 Folder Path"=w328:path, "Panel Folder Path"=w332:path)
        n119 = List Folder(path=w332, pattern="*.vi", error in=w336) -> (filenames=w334:string[], error out=w335:errorcluster)  [unwired: 1 in, 2 out]
        n120 = property on="Listbox" class="LstBox (strict)"(error in=w335, "Item Names"=w334, "Value"=w325) -> (error out=w327:errorcluster)  [unwired: 1 in, 1 out]
        n121 = List Folder(path=w328, error in=w327) -> (filenames=w330:string[], error out=w329:errorcluster)  [unwired: 2 in, 2 out]
        n122 = property on="Listbox 2" class="LstBox (strict)"(error in=w329, "Item Names"=w330, "Value"=w325) -> (error out=w326:errorcluster)  [unwired: 1 in, 1 out]
        n123 = call <vilib>:"Add State(s) to Queue__jki_lib_state_machine.vi"("State(s) in (\"\")"=w338) -> ("States Out"=w337:string)  [unwired: 14 in]
      }
      frame "SubPanel: Unload" {
        n124 = invoke on="Sub Panel" class="SubPnl" method="Remove VI"(error in=w341) -> (error out=w346:errorcluster)  [unwired: 2 in, 2 out]
        n125 = call <vilib>:"Clear Errors.vi"("error in (no error)"=w346) -> ("error out"=w340:errorcluster)  [unwired: 5 in, 1 out]
        n126 = Unbundle By Name(w345) -> ("VI Ref"=w344:refnum<vi>)
        n127 = Not A Number/Path/Refnum?(number/path/refnum=w344) -> (NaN/Path/Refnum?=w343:bool)
        n128 = case shown="False" w343 {
          tunnel: w340 -> [w357 w358]
          tunnel: [w353 w358] -> w342
          tunnel: w344 -> [w354 _]
          frame False {
            n129 = invoke class="VI (strict)" method="Ctrl Val.Set"(reference=w354, error in=w357, "Control Name"="OK", "Value"=TRUE) -> (reference out=w350:refnum<vi>, error out=w352:errorcluster)  [unwired: 1 in, 3 out]
            n130 = call-by-ref "Wait On Asynchronous Call"(reference=w350, error in=w352) -> (reference out=w349:refnum<vi>, error out=w351:errorcluster)  [unwired: 12 in]
            n131 = Close Reference(reference=w349, error in (no error)=w351) -> (error out=w353:errorcluster)
          }
          frame True {
          }
        }
        n132 = call <vilib>:"Clear Errors.vi"("error in (no error)"=w342) -> ("error out"=w339:errorcluster)  [unwired: 5 in, 1 out]
        n133 = call <vilib>:"Add State(s) to Queue__jki_lib_state_machine.vi"("State(s) in (\"\")"=w348) -> ("States Out"=w347:string)  [unwired: 14 in]
      }
      frame "SubPanel: Load" {
        n134 = Unbundle By Name(w366) -> ("VI Ref"=w364:refnum<vi>, "Panel Folder Path"=w368:path, "VI Name"=w367:string, "Time lapse(sec)"=w361:u32)
        n135 = Multiply(x=w361, y=u32 1000) -> (x*y=w359:u32)
        n136 = flat-sequence {
          tunnel: w363 -> [w373]
          tunnel: [w373] -> w362
          tunnel: w359 -> [w372]
          frame #0 {
            n137 = Wait (ms)(milliseconds to wait=w372) -> ()  [unwired: 1 out]
          }
        }
        n138 = case shown="Default" w367 {
          selector: w367 -> [_ w385]
          tunnel: [w375 w381] -> w369
          tunnel: w362 -> [w375 w380]
          tunnel: w368 -> [_ w386]
          tunnel: w366 -> [w374 w384]
          tunnel: [w374 w383] -> w365
          tunnel: w364 -> [_ w376]
          frame "" {
          }
          frame Default {
            n139 = Build Path(base path=w386, name or relative path=w385) -> (appended path=w378:path)
            n140 = File/Directory Info(path=w378, error in=w380) -> (path out=w377:path, error out=w379:errorcluster)  [unwired: 5 out]
            n141 = case shown="No Error" w379 {
              selector: w379 -> [w394 w397]
              tunnel: [w388 _] -> w382
              tunnel: [w390 w396] -> w381
              tunnel: w377 -> [w393 _]
              tunnel: w376 -> [w392 _]
              frame No Error {
                n142 = Open VI Reference(type specifier VI Refnum (for type only)=w392, vi path=w393, options=256, error in (no error)=w394) -> (vi reference=w389:refnum<vi>, error out=w395:errorcluster)  [unwired: 2 in]
                n143 = invoke on="Sub Panel" class="SubPnl" method="Insert VI"(error in=w395, "VI Ref"=w389) -> (error out=w391:errorcluster)  [unwired: 2 in, 3 out]
                n144 = call-by-ref "Start Asynchronous Call"(reference=w389, error in=w391) -> (reference out=w388:refnum<vi>, error out=w390:errorcluster)  [unwired: 12 in]
              }
              frame Error {
                n145 = call <vilib>:"Clear Errors.vi"("error in (no error)"=w397) -> ("error out"=w396:errorcluster)  [unwired: 5 in, 1 out]
              }
            }
            n146 = Bundle By Name(cluster=w384, "VI Ref"=w382) -> (w383:T8)
          }
        }
        n147 = call <vilib>:"Add State(s) to Queue__jki_lib_state_machine.vi"("State(s) in (\"\")"=w371) -> ("States Out"=w370:string)  [unwired: 14 in]
      }
      frame "SubPanel 2: Unload" {
        n148 = invoke on="Sub Panel 2" class="SubPnl" method="Remove VI"(error in=w403) -> (error out=w401:errorcluster)  [unwired: 2 in, 2 out]
        n149 = Unbundle By Name(w402) -> ("Panel 2 VI ref"=w399:refnum<vi>)
        n150 = Not A Number/Path/Refnum?(number/path/refnum=w399) -> (NaN/Path/Refnum?=w398:bool)
        n151 = case shown="True" w398 {
          tunnel: w399 -> [w407 _]
          tunnel: w401 -> [w406 w408]
          tunnel: [w405 w408] -> w400
          frame False {
            n152 = Close Reference(reference=w407, error in (no error)=w406) -> (error out=w405:errorcluster)
          }
          frame True {
          }
        }
      }
      frame "SubPanel 2: Load" {
        n153 = Unbundle By Name(w410) -> ("Panel 2 Folder Path"=w416:path, "VI Name"=w417:string)
        n154 = Build Path(base path=w416, name or relative path=w417) -> (appended path=w415:path)
        n155 = Open VI Reference(vi path=w415, error in (no error)=w413) -> (vi reference=w411:refnum<vi>, error out=w414:errorcluster)  [unwired: 4 in]
        n156 = invoke on="Sub Panel 2" class="SubPnl" method="Insert VI"(error in=w414, "VI Ref"=w411) -> (error out=w412:errorcluster)  [unwired: 2 in, 3 out]
        n157 = Bundle By Name(cluster=w410, "Panel 2 VI ref"=w411) -> (w409:T8)
      }
      frame "---------------Run------------" {
      }
      frame "Run VI" {
        n158 = Unbundle By Name(w424) -> ("Panel 2 VI ref"=w430:refnum<vi>)
        n159 = invoke class="VI" method="Run VI"(reference=w430, error in=w429, "Wait until done"=FALSE ("Wait Until Done"), "Auto Dispose Ref"=FALSE ("Auto Dispose Reference")) -> (reference out=w425:refnum<vi>, error out=w426:errorcluster)  [unwired: 1 in, 3 out]
        n160 = Bundle By Name(cluster=w424, "Panel 2 VI ref"=w425, "VI Running?"=TRUE) -> (w423:T8)
      }
      frame "---------- New Category ----------" {
        # "Template Separator\n(You can make a copy of, or modify, this frame)"
        n161 = call <vilib>:"Add State(s) to Queue__jki_lib_state_machine.vi"("State(s) in (\"\")"=w435) -> ("States Out"=w434:string)  [unwired: 14 in]
      }
      frame "New Category: 2" {
        # "Your code here.\n(You can make a copy of, or modify, this frame)"
        n162 = call <vilib>:"Add State(s) to Queue__jki_lib_state_machine.vi"("State(s) in (\"\")"=w439) -> ("States Out"=w438:string)  [unwired: 14 in]
      }
    }
  }
